vi "PAN.vi"(10 "ConfigFile in":path=path "<Not A Path>") -> ()   [LabVIEW 2016]
uses:
  private/vis/PAN_actionsSTruct.ctl
  Modules/DBSHAND/private/vis/DatabaseHand_RefNum.ctl
  Modules/DBSHAND/private/vis/DatabaseHand_Element_Set(string).vi
  Modules/DBSHAND/private/vis/DatabaseHand_Element_Set(path).vi
  Modules/DBSHAND/private/vis/DatabaseHand_Element_Get(bool).vi
panel:
  out "cinfo":string
  in  "aftexpmacro":string
  in  "expmacro":string
  in  "shutdown":string
  in  "commpath":path=path "/_COMMPATH_"
  in  "add id":bool
  out "Modules":string[](array[string])
  out "Translations":string[][](array[string])
  in  "modpath def":path=path "/_MODPATH_"
  in  "logfile":path=path "/_LOGPATH_"
  in  "log":bool
  in  "macrodir":path=path "<Not A Path>"
  in  "cmds2exec":string
  in  "errnopath":path
  in  "cmds":string
  out "DHE_DBSRef":T1
  in  "Modules":string[](array[string])=["BUFMGR"]
  in  "opencom":bool
  in  "logs":path=path "/_LOGPATH_"
  in  "configs":path=path "/_CONFPATH_"
  in  "modpath":path=path "/_MODPATH_"
  in  "ID":string
  out "init timeout":i32
  out "command":string
  in  "comsmod":string
  in  "ConfigVariables":string[][](table)=[["NetComms", "module", "PAN.vi", "comsmod", "NONE", "STR"], ["NetComms", "openpanel", "PAN.vi", "opencom", "FALSE", "BOOL"], ["PAN", "id", "PAN.vi", "ID", "NONE", "STR"], ["PAN", "modules", "PAN.vi", "modpath", "NONE", "PATH"], ["PAN", "configs", "PAN.vi", "configs", "", "PATH"], ["PAN", "logs", "PAN.vi", "logs", "", "PATH"], ["PAN", "common", "PAN.vi", "commpath", "", "PATH"], ["PAN", "commands", "PAN.vi", "cmds", "", "STR"], ["PAN", "macrodir", "PAN.vi", "macrodir", "", "PATH"], ["PAN", "autoexec", "PAN.vi", "cmds2exec", "", "STR"], ["PAN", "shutdown", "PAN.vi", "shutdown", "", "STR"], ["PAN", "beforeexp", "PAN.vi", "expmacro", "", "STR"], ["PAN", "afterexp", "PAN.vi", "aftexpmacro", "", "STR"], ["PAN", "errno", "PAN.vi", "errnopath", "", "PATH"], ["LOG", "file", "PAN.vi", "logfile", "", "PATH"], ["LOG", "log", "PAN.vi", "log", "", "BOOL"]]
  out "ConfigFile":path=path "/home/ArcVIEW/Modules/TCSP60/config/TCSP60_Default.cfg"
  in  "ModuleName":string="PAN"
  in  "action struct":T2
  out "response":string
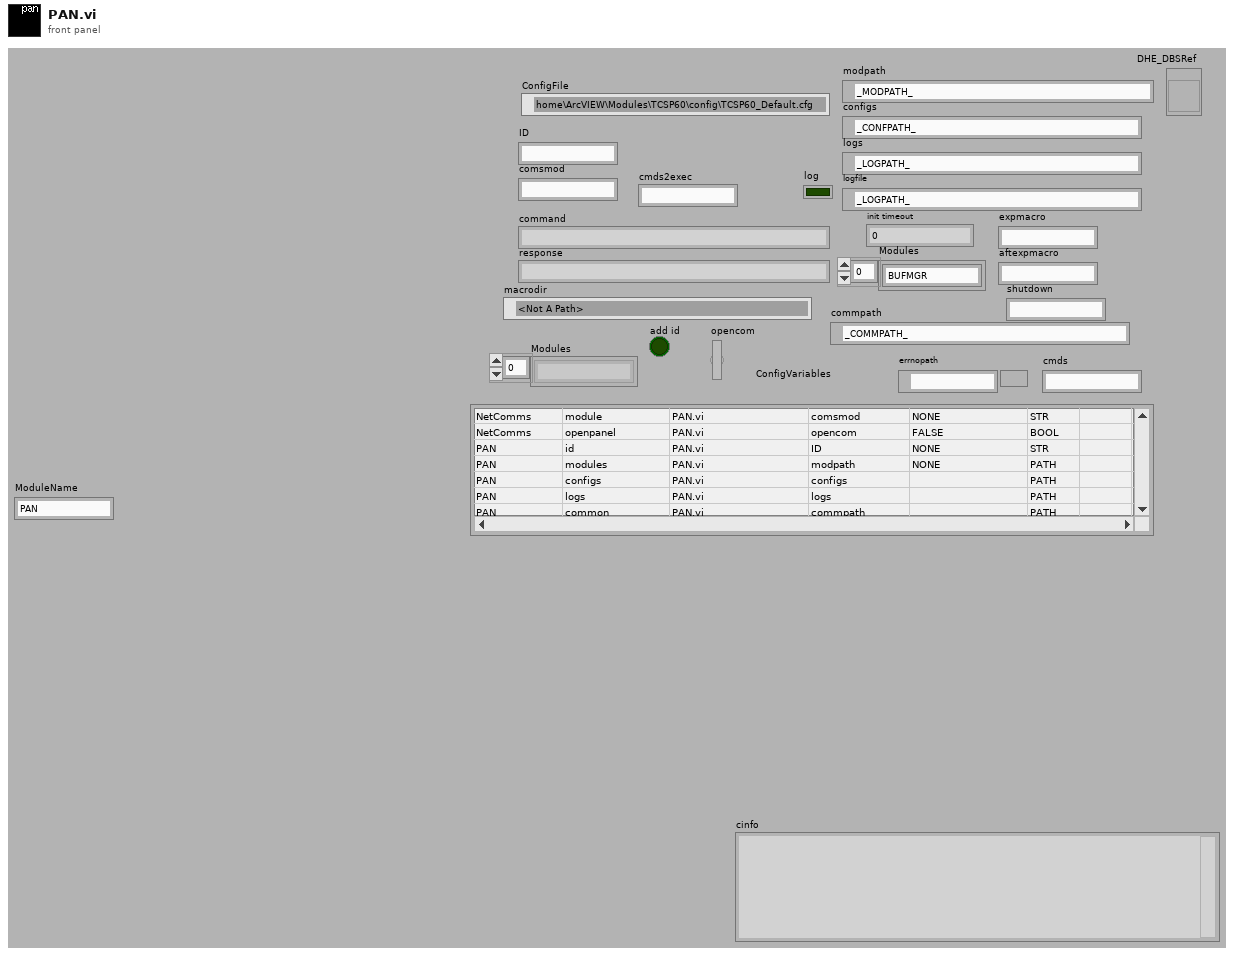
[diagram p1: front panel]
types:
  T1 = typedef "DatabaseHand_RefNum.ctl" = refnum<vi>
  T2 = typedef "PAN_actionsSTruct.ctl" = cluster{"command":string, "timeout":u32}
  T3 = typedef "PAN_cmdStruct.ctl" = cluster{"command":string, "resp Q":refnum<queue>}
  T4 = enum16{"add", "delete", "clean", "shutdown", "hold", "continue", "modify"}
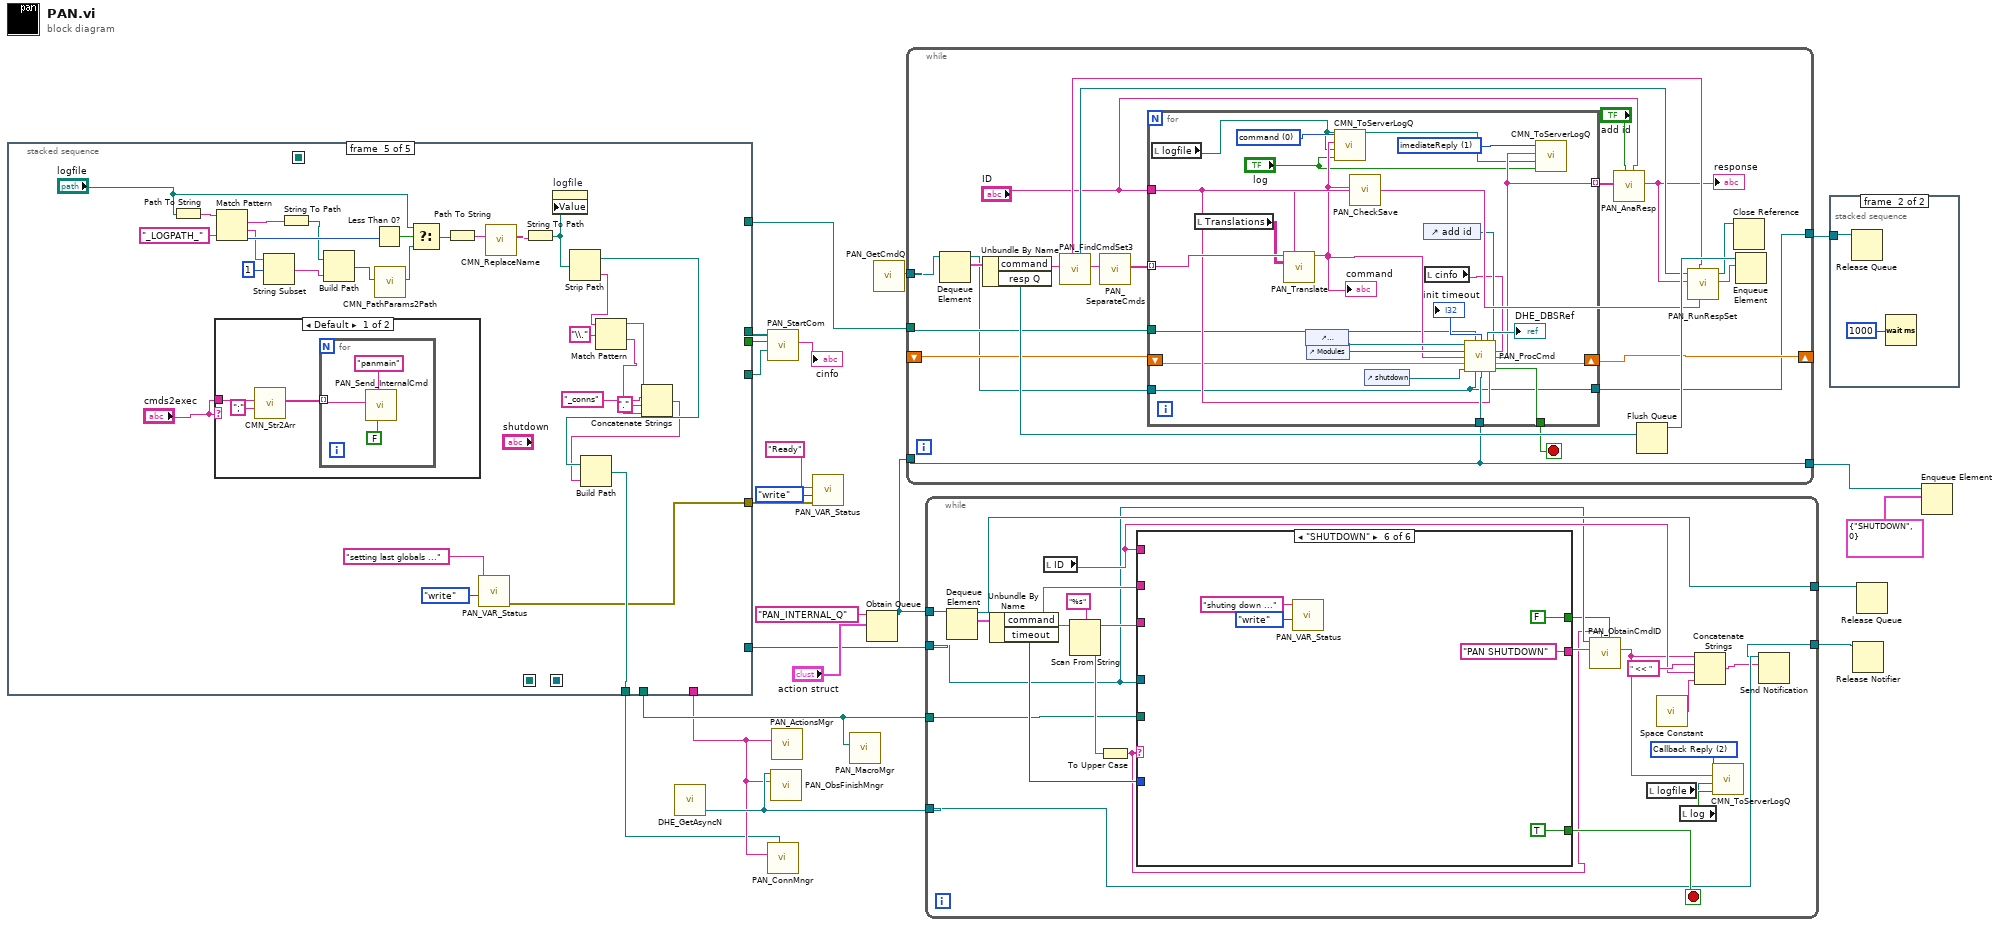
[diagram p0: block diagram]
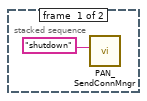
[diagram p2: hidden frame]
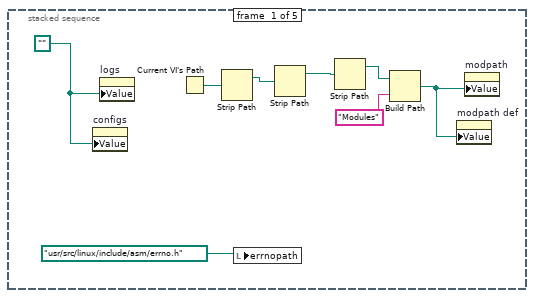
[diagram p3: hidden frame]
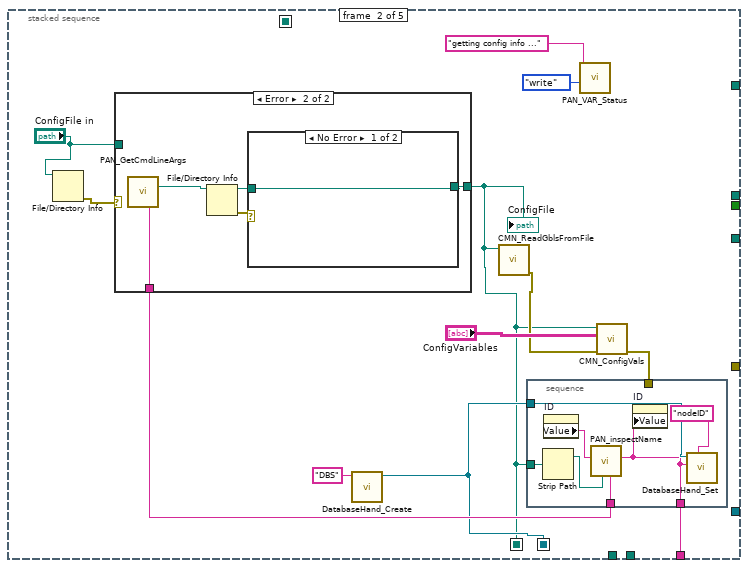
[diagram p4: hidden frame]
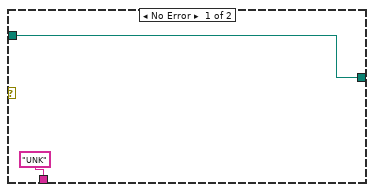
[diagram p5: hidden frame]
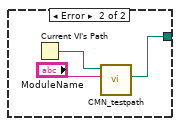
[diagram p6: hidden frame]
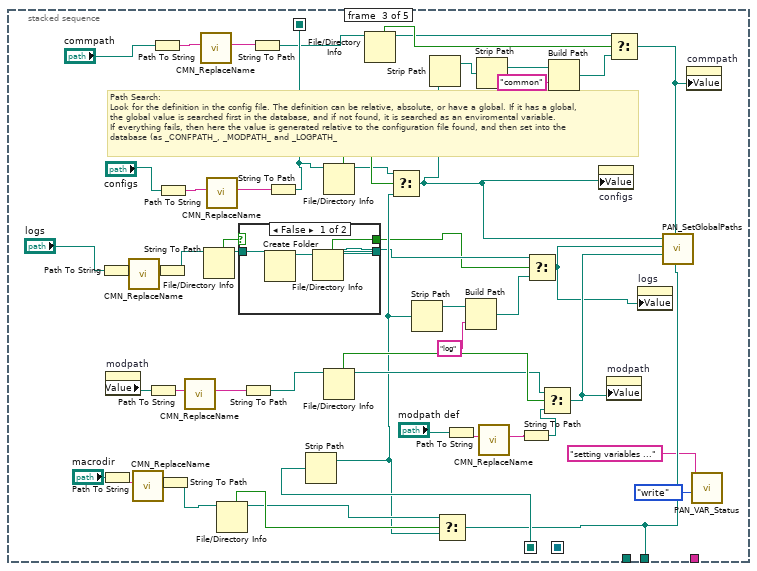
[diagram p7: hidden frame]
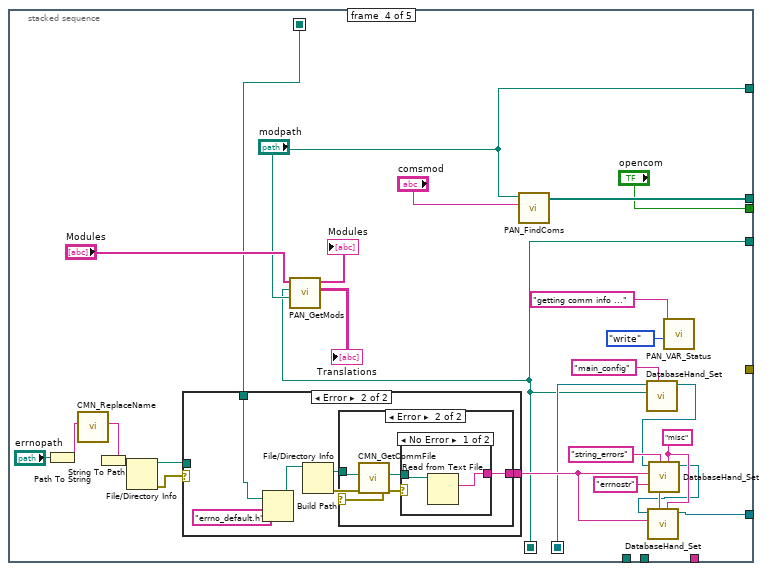
[diagram p9: hidden frame]
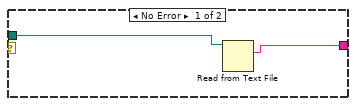
[diagram p10: hidden frame]
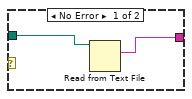
[diagram p11: hidden frame]
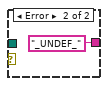
[diagram p12: hidden frame]
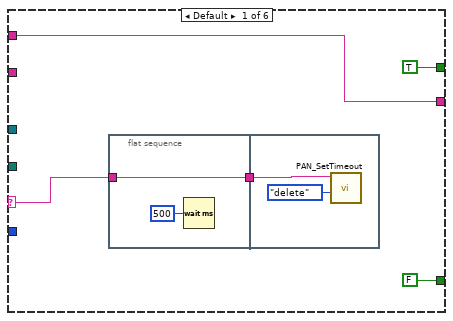
[diagram p14: hidden frame]
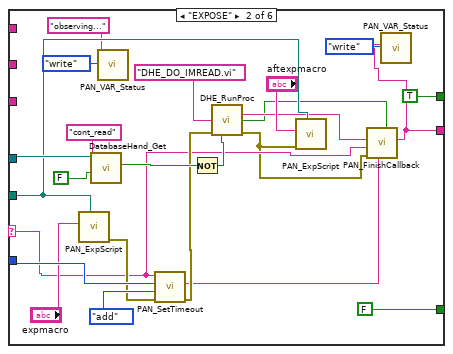
[diagram p15: hidden frame]
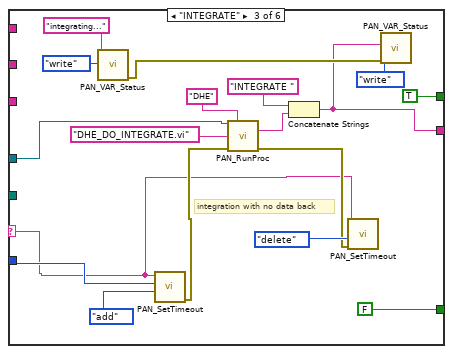
[diagram p16: hidden frame]
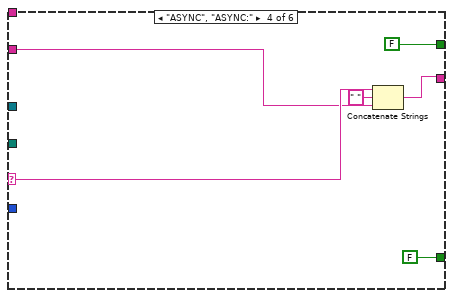
[diagram p17: hidden frame]
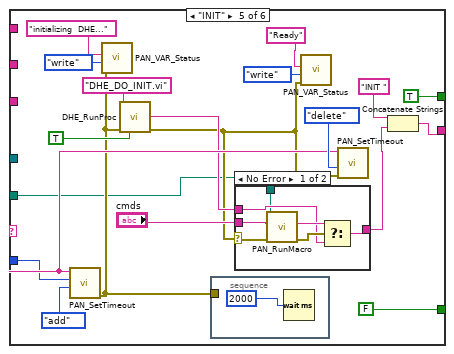
[diagram p18: hidden frame]
diagram:
  n1 = stacked-sequence {
    seq-local: [_ w34 _ _ _] -> [_ _ w110 w119 _]
    seq-local: [_ _ w96 _ _] -> [_ _ _ w129 _]
    seq-local: [_ w35 _ _ _] -> [_ _ _ w122 _]
    tunnel: [_ _ _ w144 _] -> w9
    tunnel: [_ _ _ w119 _] -> w12
    tunnel: [_ _ _ "modpath" _] -> w14
    tunnel: [_ _ _ "opencom" _] -> w13
    tunnel: [_ _ w63 _ _] -> w11
    tunnel: [_ _ _ w130 _] -> w8
    tunnel: [_ w33 _ _ _] -> w5
    tunnel: [_ _ _ _ w165] -> w4
    tunnel: [_ _ _ _ w162] -> w3
    frame #0 {
      w30 = path ""
      n2 = property on="configs" class="Path"("Value"=w30) -> ()  [unwired: 2 in, 2 out]
      n3 = property on="logs" class="Path"("Value"=w30) -> ()  [unwired: 2 in, 2 out]
      n4 = Current VI's Path() -> (path=w29:path)
      n5 = Strip Path(path=w29) -> (stripped path=w28:path)  [unwired: 1 out]
      n6 = local write "errnopath"(path "/usr/src/linux/include/asm/errno.h" ("errnopath")) -> ()
      n7 = Strip Path(path=w28) -> (stripped path=w27:path)  [unwired: 1 out]
      n8 = Strip Path(path=w27) -> (stripped path=w26:path)  [unwired: 1 out]
      n9 = Build Path(base path=w26, name or relative path="Modules") -> (appended path=w23:path)
      n10 = property on="modpath def" class="Path"("Value"=w23) -> ()  [unwired: 2 in, 2 out]
      n11 = property on="modpath" class="Path"("Value"=w23) -> ()  [unwired: 2 in, 2 out]
    }
    frame #1 {
      n12 = File/Directory Info(path="ConfigFile in") -> (error out=w40:errorcluster)  [unwired: 1 in, 6 out]
      n13 = case shown="Error" w40 {
        tunnel: [w51 w53] -> w34
        tunnel: "ConfigFile in" -> [w51 _]
        tunnel: ["UNK" ("cmdlineapp") w52] -> w37
        frame No Error {
        }
        frame Error {
          n14 = call "PAN_GetCmdLineArgs.vi"() -> ("configpath"=w56:path, "cmdlineapp"=w52:string)  [unwired: 14 out]
          n15 = File/Directory Info(path=w56) -> (path out=w54:path, error out=w55:errorcluster)  [unwired: 1 in, 5 out]
          n16 = case shown="No Error" w55 {
            tunnel: [w57 w58] -> w53
            tunnel: w54 -> [w57 _]
            frame No Error {
            }
            frame Error {
              n17 = Current VI's Path() -> (path=w60:path)
              n18 = call "CMN_testpath.vi"("ModuleName"="ModuleName", "caller Path"=w60) -> ("ConfigFile"=w58:path)  [unwired: 1 in, 8 out]
            }
          }
        }
      }
      "ConfigFile" <- w34
      n19 = call "DatabaseHand_Create.vi"("Name"="DBS") -> ("Database RefNum out"=w35:T1)  [unwired: 1 in, 9 out]
      n20 = call "CMN_ReadGblsFromFile.vi"("configuration file path"=w34) -> ("error out"=w41:errorcluster)  [unwired: 2 in, 8 out]
      n21 = call "PAN_VAR_Status.vi"("action"=enum16{"read", "write", "set_ref"}."write", "status in"="getting config info ...") -> ()  [unwired: 2 in, 8 out]
      n22 = call "CMN_ConfigVals.vi"("error in (no error)"=w41, "ConfigVariables"="ConfigVariables", "configuration file path"=w34) -> ("error out"=w38:errorcluster)  [unwired: 1 in, 7 out]
      n23 = stacked-sequence {
        tunnel: w38 -> [_]
        tunnel: w37 -> [w48]
        tunnel: w35 -> [w46]
        tunnel: w34 -> [w45]
        tunnel: [w43] -> w33
        frame #0 {
          n24 = Strip Path(path=w45) -> (stripped path=w44:path)  [unwired: 1 out]
          n25 = property on="ID" class="Str"() -> ("Value"=w49:string)  [unwired: 2 in, 2 out]
          n26 = call "PAN_inspectName.vi"("cmdline name"=w48, "pan config dir"=w44, "name in"=w49) -> ("name out"=w43:string)  [unwired: 1 in, 7 out]
          n27 = property on="ID" class="Str"("Value"=w43) -> ()  [unwired: 2 in, 2 out]
          n28 = call-poly "DatabaseHand_Set.vi"("name"="nodeID", "value"=w43, "Database RefNum in"=w46) -> ()  [unwired: 5 in, 4 out]
        }
      }
    }
    frame #2 {
      # "Path Search:\nLook for the definition in the config file. The definition can be relative, absolute, or have a global. If it has a global,\nthe global value is searched first in the database, and if not found, it is searched as an enviromental variable.\nIf everything fails, then here the value is generated relative to the configuration file found, and then set into the\ndatabase (as _CONFPATH_, _MODPATH_ and _LOGPATH_"
      n29 = Path To String(path="logs") -> (string=w95:string)
      n30 = Path To String(path="macrodir") -> (string=w91:string)
      n31 = property on="modpath" class="Path"() -> ("Value"=w88:path)  [unwired: 2 in, 2 out]
      n32 = call "CMN_ReplaceName.vi"("name in"=w95) -> ("name out"=w93:string)  [unwired: 1 in, 9 out]
      n33 = call "CMN_ReplaceName.vi"("name in"=w91) -> ("name out"=w90:string)  [unwired: 1 in, 9 out]
      n34 = Path To String(path=w88) -> (string=w87:string)
      n35 = Path To String(path="commpath") -> (string=w75:string)
      n36 = String To Path(string=w93) -> (path=w80:path)
      n37 = Path To String(path="configs") -> (string=w99:string)
      n38 = String To Path(string=w90) -> (path=w89:path)
      n39 = call "CMN_ReplaceName.vi"("name in"=w87) -> ("name out"=w86:string)  [unwired: 1 in, 9 out]
      n40 = call "CMN_ReplaceName.vi"("name in"=w75) -> ("name out"=w73:string)  [unwired: 1 in, 9 out]
      n41 = File/Directory Info(path=w80) -> (path out=w78:path, directory=w79:bool)  [unwired: 1 in, 5 out]
      n42 = call "CMN_ReplaceName.vi"("name in"=w99) -> ("name out"=w97:string)  [unwired: 1 in, 9 out]
      n43 = File/Directory Info(path=w89) -> (path out=w111:path, directory=w112:bool)  [unwired: 1 in, 5 out]
      n44 = case shown="False" w79 {
        selector: w79 -> [_ w117]
        tunnel: w78 -> [w116 w118]
        tunnel: [w113 w118] -> w77
        tunnel: [w114 w117] -> w76
        frame False {
          n45 = Create Folder(path (use dialog)=w116) -> (created path=w115:path)  [unwired: 1 in, 3 out]
          n46 = File/Directory Info(path=w115) -> (path out=w113:path, directory=w114:bool)  [unwired: 1 in, 5 out]
        }
        frame True {
        }
      }
      n47 = String To Path(string=w86) -> (path=w85:path)
      n48 = String To Path(string=w73) -> (path=w72:path)
      n49 = String To Path(string=w97) -> (path=w96:path)
      n50 = Strip Path(path=w110) -> (stripped path=w100:path)  [unwired: 1 out]
      n51 = File/Directory Info(path=w96) -> (path out=w108:path, directory=w109:bool)  [unwired: 1 in, 5 out]
      n52 = File/Directory Info(path=w85) -> (path out=w103:path, directory=w104:bool)  [unwired: 1 in, 5 out]
      n53 = File/Directory Info(path=w72) -> (path out=w70:path, directory=w71:bool)  [unwired: 1 in, 5 out]
      n54 = Select(t=w108, s=w109, f=w100) -> (s? t:f=w69:path)
      n55 = Strip Path(path=w100) -> (stripped path=w107:path)  [unwired: 1 out]
      n56 = Strip Path(path=w69) -> (stripped path=w68:path)  [unwired: 1 out]
      n57 = Select(t=w111, s=w112, f=w100) -> (s? t:f=w63:path)
      n58 = Path To String(path="modpath def") -> (string=w83:string)
      n59 = Build Path(base path=w107, name or relative path="log") -> (appended path=w105:path)
      n60 = Strip Path(path=w68) -> (stripped path=w67:path)  [unwired: 1 out]
      n61 = call "CMN_ReplaceName.vi"("name in"=w83) -> ("name out"=w82:string)  [unwired: 1 in, 9 out]
      n62 = String To Path(string=w82) -> (path=w81:path)
      n63 = Select(t=w77, s=w76, f=w105) -> (s? t:f=w101:path)
      n64 = Select(t=w103, s=w104, f=w81) -> (s? t:f=w102:path)
      n65 = Build Path(base path=w67, name or relative path="common") -> (appended path=w65:path)
      n66 = property on="configs" class="Path"("Value"=w69) -> ()  [unwired: 2 in, 2 out]
      n67 = property on="modpath" class="Path"("Value"=w102) -> ()  [unwired: 2 in, 2 out]
      n68 = Select(t=w70, s=w71, f=w65) -> (s? t:f=w64:path)
      n69 = property on="logs" class="Path"("Value"=w101) -> ()  [unwired: 2 in, 2 out]
      n70 = call "PAN_SetGlobalPaths.vi"("macro in"=w63, "common in"=w64, "modules in"=w102, "logs in"=w101, "configs in"=w69) -> ()  [unwired: 7 out]
      n71 = property on="commpath" class="Path"("Value"=w64) -> ()  [unwired: 2 in, 2 out]
      n72 = call "PAN_VAR_Status.vi"("action"=enum16{"read", "write", "set_ref"}."write", "status in"="setting variables ...") -> ()  [unwired: 2 in, 8 out]
    }
    frame #3 {
      w135 = "misc" ("group")
      n73 = Path To String(path="errnopath") -> (string=w127:string)
      n74 = call "CMN_ReplaceName.vi"("name in"=w127) -> ("name out"=w126:string)  [unwired: 1 in, 9 out]
      n75 = String To Path(string=w126) -> (path=w125:path)
      n76 = File/Directory Info(path=w125) -> (path out=w136:path, error out=w137:errorcluster)  [unwired: 1 in, 5 out]
      n77 = case shown="Error" w137 {
        tunnel: w136 -> [w146 _]
        tunnel: [w145 w148] -> w133
        tunnel: w129 -> [_ w147]
        frame No Error {
          n78 = Read from Text File(file (use dialog)=w146) -> (text=w145:string)  [unwired: 1 in, 5 out]
        }
        frame Error {
          n79 = Build Path(base path=w147, name or relative path="errno_default.h") -> (appended path=w149:path)
          n80 = File/Directory Info(path=w149) -> (path out=w150:path, error out=w151:errorcluster)  [unwired: 1 in, 5 out]
          n81 = case shown="Error" w151 {
            tunnel: w150 -> [w154 w157]
            tunnel: [w153 w158] -> w148
            frame No Error {
              n82 = Read from Text File(file (use dialog)=w154) -> (text=w153:string)  [unwired: 1 in, 5 out]
            }
            frame Error {
              n83 = call "CMN_GetCommFile.vi"("path in"=w157) -> ("error out"=w156:errorcluster, "path out"=w155:path)  [unwired: 1 in, 8 out]
              n84 = case shown="No Error" w156 {
                tunnel: [w159 "_UNDEF_"] -> w158
                tunnel: w155 -> [w160 _]
                frame No Error {
                  n85 = Read from Text File(file (use dialog)=w160) -> (text=w159:string)  [unwired: 1 in, 5 out]
                }
                frame Error {
                }
              }
            }
          }
        }
      }
      n86 = call "PAN_GetMods.vi"("Mods dir"="modpath", "configuration file path"=w119, "Mods In"="Modules") -> ("Translations"=→"Translations":string[][], "Mods Out"=→"Modules":string[])  [unwired: 7 out]
      n87 = call "PAN_FindComs.vi"("comsmod"="comsmod", "modules"="modpath") -> ("coms to run"=w144:path[])  [unwired: 9 out]
      n88 = call-poly "DatabaseHand_Set.vi"("name"="main_config" ("value"), "value"=w119, "Database RefNum in"=w122) -> ("Database RefNum out"=w121:T1)  [unwired: 5 in, 3 out]
      n89 = call-poly "DatabaseHand_Set.vi"("group"=w135, "name"="string_errors", "value"=w133, "Database RefNum in"=w121) -> ("Database RefNum out"=w132:T1)  [unwired: 4 in, 3 out]
      n90 = call-poly "DatabaseHand_Set.vi"("group"=w135, "name"="errnostr", "value"=w133, "Database RefNum in"=w132) -> ("Database RefNum out"=w130:T1)  [unwired: 4 in, 3 out]
      n91 = call "PAN_VAR_Status.vi"("action"=enum16{"read", "write", "set_ref"}."write", "status in"="getting comm info ...") -> ()  [unwired: 2 in, 8 out]
    }
    frame #4 {
      n92 = Path To String(path="logfile") -> (string=w187:string)
      n93 = case shown="Default" "cmds2exec" {
        tunnel: "cmds2exec" -> [w193 _]
        frame Default {
          n94 = call "CMN_Str2Arr.vi"("separator"=";", "string in"=w193) -> ("Array out"=w192:string[])  [unwired: 2 in, 7 out]
          n95 = for {
            tunnel: w192 -> [w195] mode=indexing
            n96 = call "PAN_Send_InternalCmd.vi"("wait response"=FALSE, "taskID"="panmain", "command"=w195) -> ()  [unwired: 2 in, 7 out]
          }
        }
        frame "", " ", "none" {
        }
      }
      n97 = Match Pattern(string=w187, regular expression="_LOGPATH_") -> (match substring=w182:string, after substring=w177:string, offset past match=w185:i32)  [unwired: 2 out]
      n98 = String Subset(string=w177, offset (0)=1) -> (substring=w175:string)  [unwired: 1 out]
      n99 = String To Path(string=w182) -> (path=w181:path)
      n100 = Build Path(base path=w181, name or relative path=w175) -> (appended path=w180:path)
      n101 = Less Than 0?(x=w185) -> (x < 0?=w184:bool)
      n102 = call "CMN_PathParams2Path.vi"("Path In"=w180) -> ("Path out"=w179:path)  [unwired: 2 in, 8 out]
      n103 = Select(t="logfile", s=w184, f=w179) -> (s? t:f=w183:path)
      n104 = Path To String(path=w183) -> (string=w189:string)
      n105 = call "PAN_VAR_Status.vi"("action"=enum16{"read", "write"}."write", "status in"="setting last globals ...") -> ("error out"=w162:errorcluster)  [unwired: 2 in, 7 out]
      n106 = call "CMN_ReplaceName.vi"("name in"=w189) -> ("name out"=w188:string)  [unwired: 1 in, 9 out]
      n107 = String To Path(string=w188) -> (path=w169:path)
      n108 = property on="logfile" class="Path"("Value"=w169) -> ()  [unwired: 2 in, 2 out]
      n109 = Strip Path(path=w169) -> (stripped path=w167:path, name=w168:string)
      n110 = Match Pattern(string=w168, regular expression="\\.") -> (before substring=w171:string, after substring=w164:string)  [unwired: 3 out]
      n111 = Concatenate Strings(w171, "_conns" ("string"), "." ("string"), w164) -> (w166:string)
      n112 = Build Path(base path=w167, name or relative path=w166) -> (appended path=w165:path)
    }
  }
  n113 = call "DHE_GetAsyncN.vi"() -> ("asyncN"=w6:refnum<notifier>)  [unwired: 11 out]
  n114 = call "PAN_StartCom.vi"("configfile"=w12, "Front Panel Window:Open"=w13, "coms to run"=w9) -> ("info"=→"cinfo":string)  [unwired: 1 in, 7 out]
  n115 = call "PAN_ConnMngr.vi"("logfile"=w4, "id"=w5) -> ()  [unwired: 10 out]
  n116 = call "PAN_ObsFinishMngr.vi"("nodeID"=w5, "notifier"=w6) -> ()  [unwired: 10 out]
  n117 = call "PAN_ActionsMgr.vi"("id"=w5) -> ()  [unwired: 1 in, 10 out]
  n118 = call "PAN_VAR_Status.vi"("error in (no error)"=w3, "action"=enum16{"read", "write", "set_ref"}."write", "status in"="Ready") -> ()  [unwired: 1 in, 8 out]
  n119 = call "PAN_MacroMgr.vi"("macrodir"=w11) -> ()  [unwired: 11 out]
  n120 = Obtain Queue(name (unnamed)="PAN_INTERNAL_Q", element data type="action struct") -> (queue out=w16:refnum<queue>)  [unwired: 3 in, 2 out]
  n121 = call "PAN_GetCmdQ.vi"() -> ("cmdQ"=w18:refnum<queue>)  [unwired: 11 out]
  n122 = while {
    shift-right: [w204] -> _
    shift-left: _ -> [w203]
    tunnel: w18 -> [w218]
    tunnel: w16 -> [w209]
    tunnel: [w197] -> w19
    tunnel: [w209] -> w15
    tunnel: w14 -> [w207]
    stop <- w208 stop-if-true
    n123 = Dequeue Element(queue=w218) -> (queue out=w198:refnum<queue>, element=w217:T3)  [unwired: 1 in, 3 out]
    n124 = Unbundle By Name(w217) -> ("command"=w211:string, "resp Q"=w216:refnum<queue>)
    n125 = call "PAN_FindCmdSet3.vi"("cmd in"=w211) -> ("native cmd out"=w206:string, "resp reference"=w214:refnum<vi>, "cmdout"=w210:string)  [unwired: 2 in, 6 out]
    n126 = call "PAN_SeparateCmds.vi"("cmd in"=w206) -> ("cmds out"=w205:string[])  [unwired: 10 out]
    n127 = for {
      tunnel: w205 -> [w238] mode=indexing
      tunnel: w209 -> [w235]
      tunnel: [w232] -> w202 mode=indexing
      tunnel: [w231] -> w208
      tunnel: "ID" -> [w229]
      tunnel: w207 -> [w228]
      tunnel: w198 -> [w222]
      shift-right: [w227] -> w204
      shift-left: w203 -> [w226]
      tunnel: [w222] -> w197
      w239 = u16 1 items=["command", "imediateReply", "Callback Reply", "Information", "none"] ("type")
      w240 = u16 0 items=["command", "imediateReply", "Callback Reply", "Information", "none"] ("type")
      n128 = local read "logfile"() -> (w220:path)
      n129 = local read "Translations"() -> (w221:string[][])
      n130 = call "PAN_Translate.vi"("command in"=w238, "app ID"=w229, "Table"=w221) -> ("command out"=w230:string)  [unwired: 1 in, 11 out]
      "command" <- w230
      n131 = control-ref of="Translations"() -> (w237:refnum<vi>)
      n132 = control-ref of="Modules"() -> (w236:refnum<vi>)
      n133 = call "CMN_ToServerLogQ.vi"("Log"="log", "file"=w220, "string"=w230, "type"=w240) -> ()  [unwired: 2 in, 5 out]
      n134 = call "PAN_CheckSave.vi"("cmd in"=w230) -> ()  [unwired: 11 out]
      n135 = control-ref of="shutdown"() -> (w224:refnum<vi>)
      n136 = control-ref of="add id"() -> (w225:refnum<vi>)
      n137 = local read "cinfo"() -> (w219:string)
      n138 = call "PAN_ProcCmd.vi"("Translations"=w237, "modpath"=w228, "addid"=w225, "Modules"=w236, "cinfo"=w219, "command in"=w230, "exp time"=w226, "shutdown"=w224, "cmdQ"=w222, "internal queue in"=w235, "nodeID"=w229) -> ("init timeout"=→"init timeout":i32, "DHE_DBSRef"=→"DHE_DBSRef":T1, "response"=w232:string, "exp time out"=w227:dbl, "shutdown"=w231:bool)
      n139 = call "CMN_ToServerLogQ.vi"("Log"="log", "file"=w220, "string"=w232, "type"=w239) -> ()  [unwired: 2 in, 5 out]
    }
    n140 = call "PAN_AnaResp.vi"("nodeID"="ID", "add id"="add id", "resp in"=w202) -> ("resp out"=w201:string)  [unwired: 8 out]
    "response" <- w201
    n141 = Flush Queue(queue=w216) -> (queue out=w215:refnum<queue>)  [unwired: 1 in, 2 out]
    n142 = call "PAN_RunRespSet.vi"("nodeID"="ID", "cmd in"=w210, "resp in"=w201, "type specifier VI Refnum (for type only)"=w214) -> ("resp out"=w213:string, "type specifier VI Refnum out"=w212:refnum<vi>)  [unwired: 1 in, 5 out]
    n143 = Close Reference(reference=w212) -> ()  [unwired: 1 in, 1 out]
    n144 = Enqueue Element(queue=w215, element=w213) -> ()  [unwired: 1 in, 4 out]
  }
  n145 = while {
    tunnel: w16 -> [w264]
    tunnel: w6 -> [w258]
    tunnel: [w256] -> w20
    tunnel: [w255] -> w17
    tunnel: w11 -> [w254]
    tunnel: w8 -> [w243]
    stop <- w259 stop-if-true
    w251 = u16 2 items=["command", "imediateReply", "Callback Reply", "Information", "none"] ("type")
    n146 = Dequeue Element(queue=w264) -> (queue out=w255:refnum<queue>, element=w261:T2)  [unwired: 1 in, 3 out]
    n147 = Unbundle By Name(w261) -> ("command"=w247:string, "timeout"=w260:u32)
    n148 = local read "ID"() -> (w246:string)
    n149 = Scan From String(format string="%s", input string=w247) -> (remaining string=w257:string, output 1=w262:string)  [unwired: 2 in, 3 out]
    n150 = To Upper Case(1:w262) -> (0:w242:string)
    n151 = case shown="\"SHUTDOWN\"" w242 {
      selector: w242 -> [w268 w282 w304 w319 w338 _]
      tunnel: w260 -> [_ w295 w314 _ w337 _]
      tunnel: [w267 w277 w301 w320 w334 "PAN SHUTDOWN" ("Result")] -> w245
      tunnel: [FALSE FALSE FALSE FALSE FALSE TRUE] -> w259
      tunnel: w257 -> [_ _ _ w318 _ _]
      tunnel: w254 -> [_ w285 _ _ w323 _]
      tunnel: w243 -> [_ w293 w300 _ _ _]
      tunnel: w247 -> [w267 _ _ _ _ _]
      tunnel: w246 -> [_ _ _ _ _ _]
      tunnel: [TRUE ("preview only") TRUE ("preview only") TRUE ("preview only") FALSE ("preview only") TRUE ("preview only") FALSE ("preview only")] -> w241
      frame Default {
        n152 = flat-sequence {
          tunnel: w268 -> [w271]
          tunnel: [w271] -> w266
          tunnel: w266 -> [w272]
          frame #0 {
            n153 = Wait (ms)(milliseconds to wait=u32 500) -> ()  [unwired: 1 out]
          }
          frame #1 {
            n154 = call "PAN_SetTimeout.vi"("action"=T4."delete", "Command"=w272) -> ()  [unwired: 2 in, 8 out]
          }
        }
      }
      frame "EXPOSE" {
        n155 = call "PAN_ExpScript.vi"("macrodir"=w285, "script"="expmacro") -> ("error out"=w287:errorcluster)  [unwired: 1 in, 8 out]
        n156 = call-poly "DatabaseHand_Get.vi"("default value"=FALSE ("wait"), "name"="cont_read", "Database RefNum in"=w293) -> ("value"=w290:bool)  [unwired: 2 in, 6 out]
        n157 = call "PAN_VAR_Status.vi"("action"=enum16{"read", "write", "set_ref"}."write", "status in"="observing...") -> ()  [unwired: 2 in, 8 out]
        n158 = call "PAN_SetTimeout.vi"("error in (no error)"=w287, "action"=T4."add", "timeout"=w295, "Command"=w282) -> ("error out"=w288:errorcluster, "obsID"=w279:string)  [unwired: 6 out]
        n159 = Not(x=w290) -> (.not. x?=w289:bool)
        n160 = call "DHE_RunProc.vi"("VItoRun"="DHE_DO_IMREAD.vi", "error in (no error)"=w288, "wait"=w289) -> ("Result"=w283:string, "wait imdone"=w280:bool, "error out"=w281:errorcluster)  [unwired: 10 out]
        n161 = call "PAN_ExpScript.vi"("macrodir"=w285, "error in (no error)"=w281, "script"="aftexpmacro") -> ()  [unwired: 9 out]
        n162 = call "PAN_FinishCallback.vi"("wait"=w280, "obsID"=w279, "error in (no error)"=w281, "Command"=w282, "response in"=w283) -> ("response out"=w277:string)  [unwired: 1 in, 5 out]
        n163 = call "PAN_VAR_Status.vi"("action"=enum16{"read", "write", "set_ref"}."write", "status in"=w277) -> ()  [unwired: 2 in, 8 out]
      }
      frame "INTEGRATE" {
        # "integration with no data back"
        n164 = call "PAN_VAR_Status.vi"("action"=enum16{"read", "write", "set_ref"}."write", "status in"="integrating...") -> ("error out"=w309:errorcluster)  [unwired: 2 in, 7 out]
        n165 = call "PAN_SetTimeout.vi"("action"=T4."add", "timeout"=w314, "Command"=w304) -> ("error out"=w305:errorcluster)  [unwired: 1 in, 7 out]
        n166 = call "PAN_RunProc.vi"("Database RefNum in"=w300, "module name"="DHE", "VItoRun"="DHE_DO_INTEGRATE.vi", "error in (no error)"=w305) -> ("Result"=w302:string, "error out"=w306:errorcluster)  [unwired: 1 in, 9 out]
        n167 = Concatenate Strings("INTEGRATE " ("string"), w302) -> (w301:string)
        n168 = call "PAN_SetTimeout.vi"("error in (no error)"=w306, "action"=T4."delete", "Command"=w304) -> ()  [unwired: 1 in, 8 out]
        n169 = call "PAN_VAR_Status.vi"("error in (no error)"=w309, "action"=enum16{"read", "write", "set_ref"}."write", "status in"=w301) -> ()  [unwired: 1 in, 8 out]
      }
      frame "ASYNC", "ASYNC:" {
        n170 = Concatenate Strings(w319, " " ("string"), w318) -> (w320:string)
      }
      frame "INIT" {
        n171 = call "PAN_SetTimeout.vi"("action"=T4."add", "timeout"=w337, "Command"=w338) -> ("error out"=w328:errorcluster)  [unwired: 1 in, 7 out]
        n172 = call "PAN_VAR_Status.vi"("error in (no error)"=w328, "action"=enum16{"read", "write", "set_ref"}."write", "status in"="initializing  DHE...") -> ()  [unwired: 1 in, 8 out]
        n173 = call "DHE_RunProc.vi"("VItoRun"="DHE_DO_INIT.vi", "error in (no error)"=w328, "wait"=TRUE) -> ("Result"=w333:string, "error out"=w324:errorcluster)  [unwired: 11 out]
        n174 = stacked-sequence {
          tunnel: w328 -> [_]
          frame #0 {
            n175 = Wait (ms)(milliseconds to wait=u32 2000) -> ()  [unwired: 1 out]
          }
        }
        n176 = case shown="No Error" w324 {
          selector: w324 -> [w349 _]
          tunnel: [w345 w350] -> w332
          tunnel: w333 -> [w346 w350]
          tunnel: w323 -> [w344 _]
          tunnel: "cmds" -> [w343 _]
          frame No Error {
            n177 = call "PAN_RunMacro.vi"("error in (no error)"=w349, "commands"=w343, "macrodir"=w344) -> ("error out"=w348:errorcluster, "response"=w347:string)  [unwired: 7 out]
            n178 = Select(t=w347, s=w348, f=w346) -> (s? t:f=w345:string)
          }
          frame Error {
          }
        }
        n179 = call "PAN_VAR_Status.vi"("error in (no error)"=w324, "action"=enum16{"read", "write", "set_ref"}."write", "status in"="Ready") -> ()  [unwired: 1 in, 8 out]
        n180 = call "PAN_SetTimeout.vi"("error in (no error)"=w324, "action"=T4."delete", "Command"=w338) -> ()  [unwired: 1 in, 8 out]
        n181 = Concatenate Strings("INIT " ("string"), w332) -> (w334:string)
      }
      frame "SHUTDOWN" {
        n182 = call "PAN_VAR_Status.vi"("action"=enum16{"read", "write", "set_ref"}."write", "status in"="shuting down ...") -> ()  [unwired: 2 in, 8 out]
      }
    }
    n183 = call "PAN_ObtainCmdID.vi"("send cmdid"=w241, "source"=w242, "resp in"=w245, "Database RefNum in"=w243) -> ("resp out"=w244:string)  [unwired: 7 out]
    n184 = local read "logfile"() -> (w252:path)
    n185 = call <vilib>:"Space Constant.vi"() -> ("String"=w248:string)
    n186 = local read "log"() -> (w253:bool)
    n187 = Concatenate Strings(w244, " << " ("string"), w246, w248) -> (w250:string)
    n188 = call "CMN_ToServerLogQ.vi"("Log"=w253, "file"=w252, "string"=w244, "type"=w251) -> ()  [unwired: 2 in, 5 out]
    n189 = Send Notification(notification=w250, notifier=w258) -> (notifier out=w256:refnum<notifier>)  [unwired: 1 in, 1 out]
  }
  n190 = stacked-sequence {
    tunnel: w19 -> [_ w357]
    frame #0 {
      n191 = call "PAN_SendConnMngr.vi"("command"="shutdown") -> ()  [unwired: 2 in, 9 out]
    }
    frame #1 {
      n192 = Release Queue(queue=w357) -> ()  [unwired: 1 in, 4 out]
      n193 = Wait (ms)(milliseconds to wait=u32 1000) -> ()  [unwired: 1 out]
    }
  }
  n194 = Release Notifier(notifier=w20) -> ()  [unwired: 1 in, 4 out]
  n195 = Release Queue(queue=w17) -> ()  [unwired: 1 in, 4 out]
  n196 = Enqueue Element(queue=w15, element=T2 {"command"="SHUTDOWN", "timeout"=0}) -> ()  [unwired: 1 in, 4 out]
